vi "test_Configure Response_Invalid Response Refnum Error.vi"(8 "error in (no error)":errorcluster, 11 "TestCase in":refnum<class "Instrument Addon Scripting API Messages Unit Tests.lvclass">) -> (0 "error out":errorcluster, 3 "TestCase out":refnum<class "Instrument Addon Scripting API Messages Unit Tests.lvclass">)   [LabVIEW 2020, in "Instrument Addon Scripting API Messages Unit Tests.lvclass"]
uses:
  Instrument Addon Scripting API Messages Unit Tests.lvclass
  APIs/Scripting API/TypeDefs/ByteCount Response Settings.ctl
  APIs/Scripting API/TypeDefs/Linked Channel.ctl
  <vilib>/NI VeriStand/Custom Device API/Custom Device Item Ref.ctl
  Instrument Addon Scripting API Messages Unit Tests.lvclass/Instrument Addon Scripting API Messages Unit Tests.ctl
  Addon/Addon Shared/SubVIs/Constants.vi
  <vilib>/NI/NI VeriStand Advanced SysDef API/_SubVIs/SysDef.Search.GUID.vi
  APIs/Scripting API/Messages/Configure Response - Byte Count.vi
  <vilib>/addons/_JKI Toolkits/VI Tester/TestCase.llb/TestCase.lvclass
  <vilib>/NI/NI VeriStand Advanced SysDef API/SysDef API/Advanced System Definition.lvlib
  Addon/Addon Shared/Instrument Addon Shared.lvlib
  APIs/Scripting API/Instrument Addon Scripting API.lvlib
  <vilib>/NI VeriStand/Custom Device API/Custom Device API.lvlib
  C:/Program Files (x86)/National Instruments/LabVIEW 2020/vi.lib/addons/_JKI Toolkits/VI Tester/TestCase.llb/TestCase.lvclass
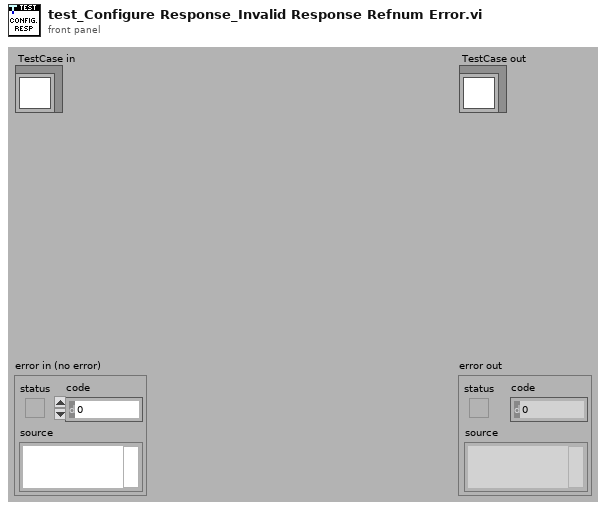
[diagram p1: front panel]
types:
  T1 = typedef "Instrument Addon Scripting API.lvlib/ByteCount Response Settings.ctl" = cluster{"Response Format":string, "Linked Channels":T2[], "Byte Count":i32, "Use Byte Count channel":bool, "Channel Refnum":T3}
  T2 = typedef "Instrument Addon Scripting API.lvlib/Linked Channel.ctl" = cluster{"Variable Name":string, "Channel Refnum":T3}
  T3 = typedef "Custom Device API.lvlib/Custom Device Item Ref.ctl" = u64
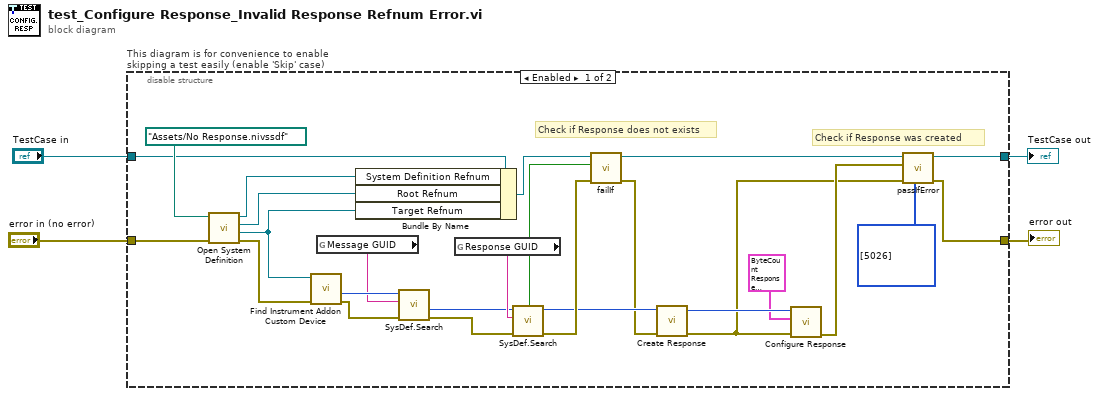
[diagram p0: block diagram]
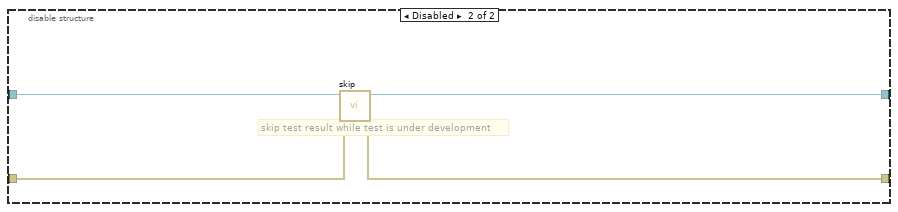
[diagram p2: hidden frame]
diagram:
  n1 = disable-structure "This diagram is for convenience to enable skipping a test easily (enable 'Skip' case)" shown="Enabled" {
    disable-tunnel: "TestCase in" -> [w16 w34]
    disable-tunnel: [w22 w32] -> w1
    disable-tunnel: [w23 w33] -> w3
    disable-tunnel: "error in (no error)" -> [w29 w31]
    frame Enabled {
      # "Check if Response was created"
      # "Check if Response does not exists"
      n2 = call "Open System Definition.vi"("error in (no error)"=w29, "System Definition File"=path "Assets/No Response.nivssdf" ("SDF file")) -> ("error out"=w28:errorcluster, "Target Refnum"=w15:refnum<k24>, "Root Refnum"=w14:refnum<k24>, "System Definition Refnum"=w13:refnum<k24>)  [unwired: 6 in]
      n3 = call "Find Instrument Addon Custom Device.vi"("error in"=w28, "target in"=w15) -> ("error out"=w20:errorcluster, "NodeID"=w21:u64)  [unwired: 7 in, 1 out]
      n4 = global read "Constants.vi" "Message GUID"() -> (w19:string)
      n5 = Bundle By Name(cluster=w16, "System Definition Refnum"=w13, "Root Refnum"=w14, "Target Refnum"=w15) -> (w12:refnum<class "Instrument Addon Scripting API Messages Unit Tests.lvclass">)
      n6 = call-poly <vilib>:"SysDef.Search.vi"("error in (no error)"=w20, "GUID"=w19, "nodeID"=w21) -> ("error out"=w18:errorcluster, "Value out"=w17:u64)  [unwired: 5 in, 2 out]
      n7 = global read "Constants.vi" "Response GUID"() -> (w27:string)
      n8 = call-poly <vilib>:"SysDef.Search.vi"("error in (no error)"=w18, "GUID"=w27, "nodeID"=w17) -> ("error out"=w25:errorcluster, "nodeID out"=w11:u64, "Found?"=w26:bool)  [unwired: 5 in, 1 out]
      n9 = call-dynamic "failIf.vi"("error in (no error)"=w25, "fail"=w26, "TestCase in"=w12) -> ("error out"=w10:errorcluster, "TestCase out"=w24:refnum<class "Instrument Addon Scripting API Messages Unit Tests.lvclass">)  [unwired: 7 in]
      n10 = call "Create Response.vi"("error in (no error)"=w10, "message refnum in"=w11) -> ("error out"=w6:errorcluster, "message refnum out"=w9:T3)  [unwired: 7 in, 1 out]
      n11 = call-poly "Configure Response.vi"("error in (no error)"=w6, "settings"=T1 {"Response Format"="[Var1]+[Var2]", "Linked Channels"=[{"Variable Name"="Var1", "Channel Refnum"=3537}, {"Variable Name"="Var2", "Channel Refnum"=3538}], "Byte Count"=32, "Use Byte Count channel"=FALSE, "Channel Refnum"=3539}, "response refnum in"=w9) -> ("error out"=w7:errorcluster)  [unwired: 7 in, 1 out]
      n12 = call-dynamic "passIfError.vi"("passing error codes (default = any error code)"=i32[] [5026], "error in (no error)"=w6, "error"=w7, "TestCase in"=w24) -> ("error out"=w23:errorcluster, "TestCase out"=w22:refnum<class "Instrument Addon Scripting API Messages Unit Tests.lvclass">)  [unwired: 6 in]
    }
    frame Disabled {
      # "skip test result while test is under development"
      n13 = call <vilib>:"skip.vi"("error in (no error)"=w31, "TestCase in"=w34) -> ("error out"=w33:errorcluster, "TestCase out"=w32:refnum<class "Instrument Addon Scripting API Messages Unit Tests.lvclass">)  [unwired: 8 in]
    }
  }
  "error out" <- w3
  "TestCase out" <- w1
